vi "Read Status.vi"() -> ()   [LabVIEW 2011, in "MGC647C.lvlib"]
doc: "This sample VI illustrates the usage of the driver toread the actual device status."
uses:
  <instrlib>/MGC647C/MGC647C.lvlib
  <userlib>/FGV_Utilities/HGF_FGV_File/Action Text File.ctl
  <userlib>/FGV_Utilities/HGF_FGV_File/HGF_FGV_File.lvlib
panel:
  out "Channels":T1(array[cluster])
  out "Instrument Firmware Revision":string
  out "Instrument Driver Revision":string
  out "Controller Code":enum16{"STD", "250", "152", "---", "652", "146"}(ring)
  out "Pressure Mode":bool
  out "Pressure Setpoint":dbl
  out "Gas Menu":i32
  in  "#Channels":i32=4
  out "Unit":T2(ring)=enum."1.0000 Pa"
  out "Actual Pressure":dbl
  in  "Serial Configuration":T3={"Baud Rate"=9600, "Parity"=0, "Data Bits"=8, "Stop Bits"=10, "Flow Control"=0} {"Flow Control" items=["None", "XON/XOFF", "RTS/CTS", "XON/XOFF & RTS/CTS", "DTR/DSR", "XON/XOFF & DTR/DSR"]; "Stop Bits" items=["1.0"=10, "1.5"=15, "2.0"=20]; "Data Bits" items=["7"=7, "8"=8]; "Parity" items=["None", "Odd", "Even", "Mark", "Space"]; "Baud Rate" items=["300"=300, "600"=600, "1200"=1200, "2400"=2400, "4800"=4800, "9600"=9600, "19200"=19200]}
  in  "VISA resource name":refnum<visa-resource-name>
  # "(C) Copyright 2012 GSI Helmholtzzentrum für Schwerionenforschung GmbH.  ALL RIGHTS RESERVED."
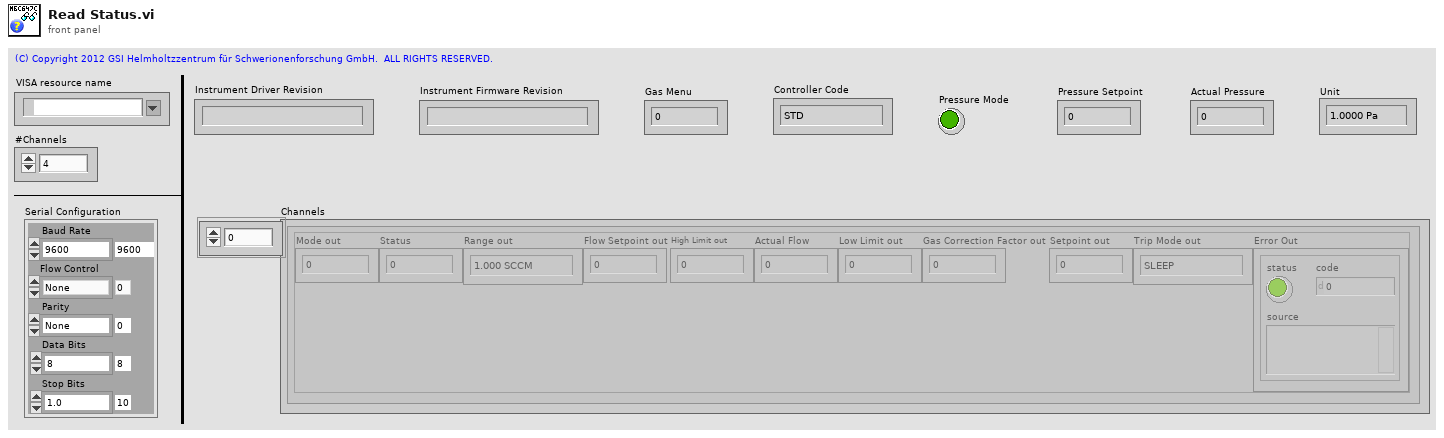
[diagram p1: front panel]
types:
  T1 = cluster{"Mode out":u16, "Status":u16, "Range out":enum16{"1.000 SCCM", "2.000 SCCM", "5.000 SCCM", "10.00 SCCM", "20.00 SCCM", "50.00 SCCM", "100.0 SCCM", "200.0 SCCM", "500.0 SCCM", "1.000 SLM", "2.000 SLM", "5.000 SLM", "10.00 SLM", "20.00 SLM", "50.00 SLM", "100.0 SLM", "200.0 SLM", "400.0 SLM", "500.0 SLM", "1.000 SCMM", "1.000 SCFH", "2.000 SCFH", "5.000 SCFH", "10.00 SCFH", "20.00 SCFH", "50.00 SCFH", "100.0 SCFH", "200.0 SCFH", "500.0 SCFH", "1.000 SCFM", "2.000 SCFM", "5.000 SCFM", "10.00 SCFM", "20.00 SCFM", "50.00 SCFM", "100.0 SCFM", "200.0 SCFM", "500.0 SCFM", "30.00 SLM", "300.0 SLM"}, "Flow Setpoint out":dbl, "High Limit out":dbl, "Actual Flow":dbl, "Low Limit out":dbl, "Gas Correction Factor out":dbl, "Setpoint out":dbl, "Trip Mode out":enum16{"SLEEP", "LIMIT", "BAND"}, "Error Out":errorcluster}[]
  T2 = enum16{"1.0000 mTorr", "10.000 mTorr", "100.00 mTorr", "1000.0 mTorr", "1.0000 Torr", "10.000 Torr", "100.00 Torr", "1000.0 Torr", "1.0000 kTorr", "10.000 kTorr", "100.00 kTorr", "1.0000 µBar", "10.000 µBar", "100.00 µBar", "1000.0 µBar", "1.0000 mBar", "10.000 mBar", "100.00 mBar", "1000.0 mBar", "1.0000 Bar", "10.000 Bar", "100.00 Bar", "1.0000 Pa", "10.000 Pa", "100.00 Pa", "1.0000 kPa", "10.000 kPa", "100.00 kPa", "1000.0 kPa"}
  T3 = cluster{"Baud Rate":u32, "Parity":u16, "Data Bits":u16, "Stop Bits":u16, "Flow Control":u16}
  T4 = enum16{"open", "replace", "create", "open or create", "replace or create", "replace or create with confirmation"}
  T5 = typedef "HGF_FGV_File.lvlib/Action Text File.ctl" = enum16{"open file", "read lines", "read characters", "write", "flush", "close file", ""}
  T6 = enum16{"1.000 SCCM", "2.000 SCCM", "5.000 SCCM", "10.00 SCCM", "20.00 SCCM", "50.00 SCCM", "100.0 SCCM", "200.0 SCCM", "500.0 SCCM", "1.000 SLM", "2.000 SLM", "5.000 SLM", "10.00 SLM", "20.00 SLM", "50.00 SLM", "100.0 SLM", "200.0 SLM", "400.0 SLM", "500.0 SLM", "1.000 SCMM", "1.000 SCFH", "2.000 SCFH", "5.000 SCFH", "10.00 SCFH", "20.00 SCFH", "50.00 SCFH", "100.0 SCFH", "200.0 SCFH", "500.0 SCFH", "1.000 SCFM", "2.000 SCFM", "5.000 SCFM", "10.00 SCFM", "20.00 SCFM", "50.00 SCFM", "100.0 SCFM", "200.0 SCFM", "500.0 SCFM", "30.00 SLM", "300.0 SLM"}
  T7 = cluster{"Mode out":u16, "Status":u16, "Range out":enum16{"1.000 SCCM", "2.000 SCCM", "5.000 SCCM", "10.00 SCCM", "20.00 SCCM", "50.00 SCCM", "100.0 SCCM", "200.0 SCCM", "500.0 SCCM", "1.000 SLM", "2.000 SLM", "5.000 SLM", "10.00 SLM", "20.00 SLM", "50.00 SLM", "100.0 SLM", "200.0 SLM", "400.0 SLM", "500.0 SLM", "1.000 SCMM", "1.000 SCFH", "2.000 SCFH", "5.000 SCFH", "10.00 SCFH", "20.00 SCFH", "50.00 SCFH", "100.0 SCFH", "200.0 SCFH", "500.0 SCFH", "1.000 SCFM", "2.000 SCFM", "5.000 SCFM", "10.00 SCFM", "20.00 SCFM", "50.00 SCFM", "100.0 SCFM", "200.0 SCFM", "500.0 SCFM", "30.00 SLM", "300.0 SLM"}, "Flow Setpoint out":dbl, "High Limit out":dbl, "Actual Flow":dbl, "Low Limit out":dbl, "Gas Correction Factor out":dbl, "Setpoint out":dbl, "Trip Mode out":enum16{"SLEEP", "LIMIT", "BAND"}, "Error Out":errorcluster}
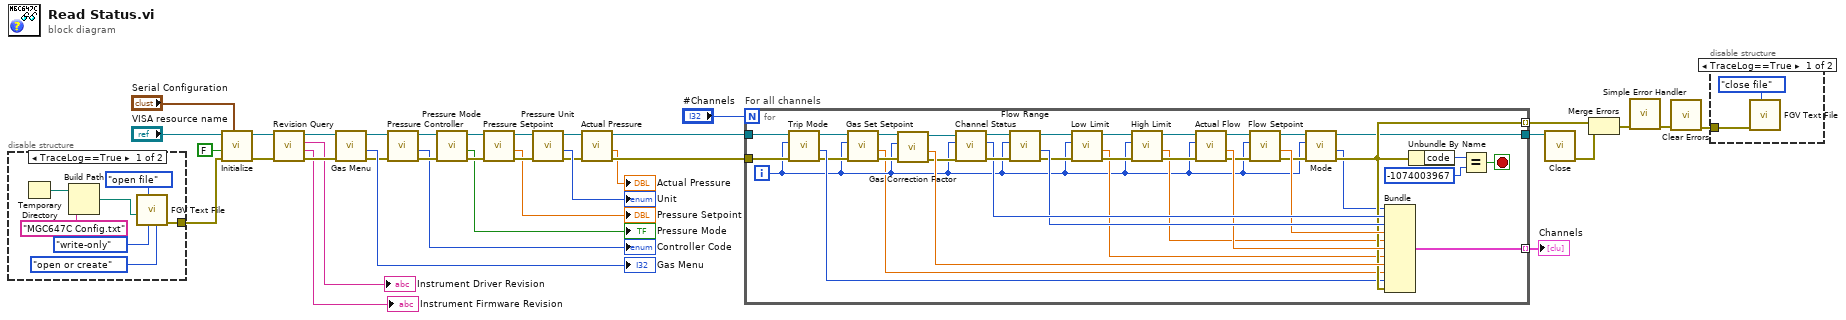
[diagram p0: block diagram]
diagram:
  n1 = disable-structure shown="TraceLog==True" {
    disable-tunnel: [w42 _] -> w1
    frame condition #0 (active) {
      n2 = Temporary Directory() -> (w39:path)
      n3 = Build Path(base path=w39, name or relative path="MGC647C Config.txt" ("file path (empty)")) -> (appended path=w37:path)
      n4 = call <userlib>:"FGV Text File.vi"("operation (0:open)"=T4."open or create", "access (0:read/write)"=enum16{"read/write", "read-only", "write-only"}."write-only", "Action"=Action_Text_File."open file", "file path (empty)"=w37) -> ("Error Out"=w42:errorcluster)  [unwired: 5 in, 2 out]
    }
    frame condition #1 {
    }
  }
  n5 = call <instrlib>:"Initialize.vi"("Serial Configuration"="Serial Configuration", "error in (no error)"=w1, "Reset (True)"=FALSE, "VISA resource name"="VISA resource name") -> ("error out"=w10:errorcluster, "VISA resource name out"=w11:refnum<visa-resource-name>)  [unwired: 6 in]
  n6 = call <instrlib>:"Revision Query.vi"("error in (no error)"=w10, "VISA resource name"=w11) -> ("error out"=w8:errorcluster, "Instrument Firmware Revision"=→"Instrument Firmware Revision":string, "Instrument Driver Revision"=→"Instrument Driver Revision":string, "VISA resource name out"=w9:refnum<visa-resource-name>)  [unwired: 6 in]
  n7 = call <instrlib>:"Gas Menu.vi"("Error In"=w8, "VISA resource name"=w9) -> ("Error Out"=w12:errorcluster, "Gas Menu out"=→"Gas Menu":i32, "dup VISA resource name"=w13:refnum<visa-resource-name>)  [unwired: 7 in]
  n8 = call <instrlib>:"Pressure Controller.vi"("Error In"=w12, "VISA resource name"=w13) -> ("Error Out"=w19:errorcluster, "Controller Code out"=→"Controller Code":enum16{"STD", "250", "152", "---", "652", "146"}, "dup VISA resource name"=w20:refnum<visa-resource-name>)  [unwired: 7 in]
  n9 = call <instrlib>:"Pressure Mode.vi"("Error In"=w19, "VISA resource name"=w20) -> ("Error Out"=w18:errorcluster, "Pressure Mode"=→"Pressure Mode":bool, "dup VISA resource name"=w21:refnum<visa-resource-name>)  [unwired: 7 in]
  n10 = call <instrlib>:"Pressure Setpoint.vi"("Error In"=w18, "VISA resource name"=w21) -> ("Error Out"=w17:errorcluster, "Pressure Setpoint out"=→"Pressure Setpoint":dbl, "dup VISA resource name"=w22:refnum<visa-resource-name>)  [unwired: 7 in]
  n11 = call <instrlib>:"Pressure Unit.vi"("Error In"=w17, "VISA resource name"=w22) -> ("Error Out"=w28:errorcluster, "Unit out"=→"Unit":T2, "dup VISA resource name"=w32:refnum<visa-resource-name>)  [unwired: 7 in]
  n12 = call <instrlib>:"Actual Pressure.vi"("Error In"=w28, "VISA resource name"=w32) -> ("Error Out"=w29:errorcluster, "Actual Pressure"=→"Actual Pressure":dbl, "dup VISA resource name"=w30:refnum<visa-resource-name>)  [unwired: 7 in]
  n13 = for "For all channels" {
    N: "#Channels" -> [_]
    tunnel: w30 -> [w52]
    tunnel: w29 -> [w51]
    tunnel: [w73] -> w5 mode=indexing
    tunnel: [w63] -> w25 mode=indexing
    tunnel: [w62] -> w34
    i -> [w45]
    stop <- w76 stop-if-true
    n14 = call <instrlib>:"Trip Mode.vi"("Error In"=w51, "Channel (0)"=w45, "VISA resource name"=w52) -> ("Error Out"=w47:errorcluster, "Trip Mode out"=w50:enum16{"SLEEP", "LIMIT", "BAND"}, "dup VISA resource name"=w49:refnum<visa-resource-name>)  [unwired: 6 in]
    n15 = call <instrlib>:"Gas Set Setpoint.vi"("Error In"=w47, "Channel (0)"=w45, "VISA resource name"=w49) -> ("Error Out"=w46:errorcluster, "Setpoint out"=w44:dbl, "dup VISA resource name"=w48:refnum<visa-resource-name>)  [unwired: 6 in]
    n16 = call <instrlib>:"Gas Correction Factor.vi"("Error In"=w46, "Channel (0)"=w45, "VISA resource name"=w48) -> ("Error Out"=w67:errorcluster, "Gas Correction Factor out"=w68:dbl, "dup VISA resource name"=w66:refnum<visa-resource-name>)  [unwired: 6 in]
    n17 = call <instrlib>:"Channel Status.vi"("Error In"=w67, "Channel (-1:Main)"=w45, "VISA resource name"=w66) -> ("Error Out"=w79:errorcluster, "Status"=w75:u16, "dup VISA resource name"=w80:refnum<visa-resource-name>)  [unwired: 5 in, 1 out]
    n18 = call <instrlib>:"Flow Range.vi"("Error In"=w79, "Channel (0)"=w45, "VISA resource name"=w80) -> ("Error Out"=w59:errorcluster, "Range out"=w74:T6, "dup VISA resource name"=w60:refnum<visa-resource-name>)  [unwired: 6 in]
    n19 = call <instrlib>:"Low Limit.vi"("Error In"=w59, "Channel (0)"=w45, "VISA resource name"=w60) -> ("Error Out"=w57:errorcluster, "Low Limit out"=w53:dbl, "dup VISA resource name"=w58:refnum<visa-resource-name>)  [unwired: 6 in]
    n20 = call <instrlib>:"High Limit.vi"("Error In"=w57, "Channel (0)"=w45, "VISA resource name"=w58) -> ("Error Out"=w55:errorcluster, "High Limit out"=w54:dbl, "dup VISA resource name"=w56:refnum<visa-resource-name>)  [unwired: 6 in]
    n21 = call <instrlib>:"Actual Flow.vi"("Error In"=w55, "Channel (0)"=w45, "VISA resource name"=w56) -> ("Error Out"=w69:errorcluster, "Actual Flow"=w72:dbl, "dup VISA resource name"=w70:refnum<visa-resource-name>)  [unwired: 6 in]
    n22 = call <instrlib>:"Flow Setpoint.vi"("Error In"=w69, "Channel (0)"=w45, "VISA resource name"=w70) -> ("Error Out"=w64:errorcluster, "Flow Setpoint out"=w71:dbl, "dup VISA resource name"=w65:refnum<visa-resource-name>)  [unwired: 6 in]
    n23 = call <instrlib>:"Mode.vi"("Error In"=w64, "Channel (0)"=w45, "VISA resource name"=w65) -> ("Error Out"=w63:errorcluster, "Mode out"=w61:u16, "dup VISA resource name"=w62:refnum<visa-resource-name>)  [unwired: 5 in, 1 out]
    n24 = Bundle("Mode out"=w61, "Status"=w75, "Range out"=w74, "Flow Setpoint out"=w71, "High Limit out"=w54, "Actual Flow"=w72, "Low Limit out"=w53, "Gas Correction Factor out"=w68, "Setpoint out"=w44, "Trip Mode out"=w50, "Error Out"=w63) -> (w73:T7)  [unwired: 1 in]
    n25 = Unbundle By Name(w63) -> ("code"=w78:i32)
    n26 = Equal?(x=w78, y=-1074003967) -> (x = y?=w76:bool)
  }
  "Channels" <- w5
  n27 = call <instrlib>:"Close.vi"("VISA resource name"=w34) -> ("error out"=w24:errorcluster)  [unwired: 10 in]
  n28 = Merge Errors(w25, w24) -> (w33:errorcluster)
  n29 = call <vilib>:"Simple Error Handler.vi"("error in (no error)"=w33) -> ("error out"=w3:errorcluster)  [unwired: 4 in, 4 out]
  n30 = call <vilib>:"Clear Errors.vi"("error in (no error)"=w3) -> ("error out"=w2:errorcluster)  [unwired: 6 in]
  n31 = disable-structure shown="TraceLog==True" {
    disable-tunnel: w2 -> [w81 _]
    frame condition #0 (active) {
      n32 = call <userlib>:"FGV Text File.vi"("Action"=Action_Text_File."close file", "Error In"=w81) -> ()  [unwired: 7 in, 3 out]
    }
    frame condition #1 {
    }
  }
